vi "KickSkillVSS.vi"(8 "error in (no error)":errorcluster, 9 "BallRef":refnum<class "Ball.lvclass">, 10 "Robot":refnum<class "Robot.lvclass">, 11 "KickSkillVSS in":refnum<class "KickSkillVSS.lvclass">) -> (0 "error out":errorcluster, 2 "Robot out":refnum<class "Robot.lvclass">, 3 "KickSkillVSS out":refnum<class "KickSkillVSS.lvclass">)   [LabVIEW 2020, in "KickSkillVSS.lvclass"]
uses:
  KickSkillVSS.lvclass
  Robot_class/Robot.lvclass
  Ball_class/Ball.lvclass
  Field_class/Field.lvclass
  Utilities_class/Utilities.lvclass
  Object_class/Object.lvclass/Object.ctl
  Ball_class/Ball.lvclass/Ball.ctl
  Robot_class/Robot.lvclass/Robot.ctl
  Object_class/Read x.vi
  Object_class/Read y.vi
  Ball_class/Read v_x.vi
  Ball_class/Read v_y.vi
  Object_class/Read pos_est_x.vi
  Object_class/Read pos_est_y.vi
  Robot_class/Write orientation.vi
panel:
  in  "Field":refnum<class "Field.lvclass">
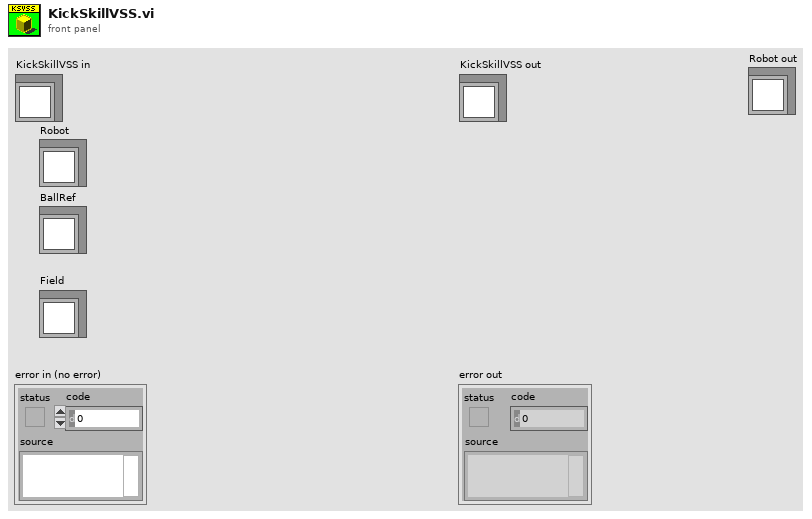
[diagram p1: front panel]
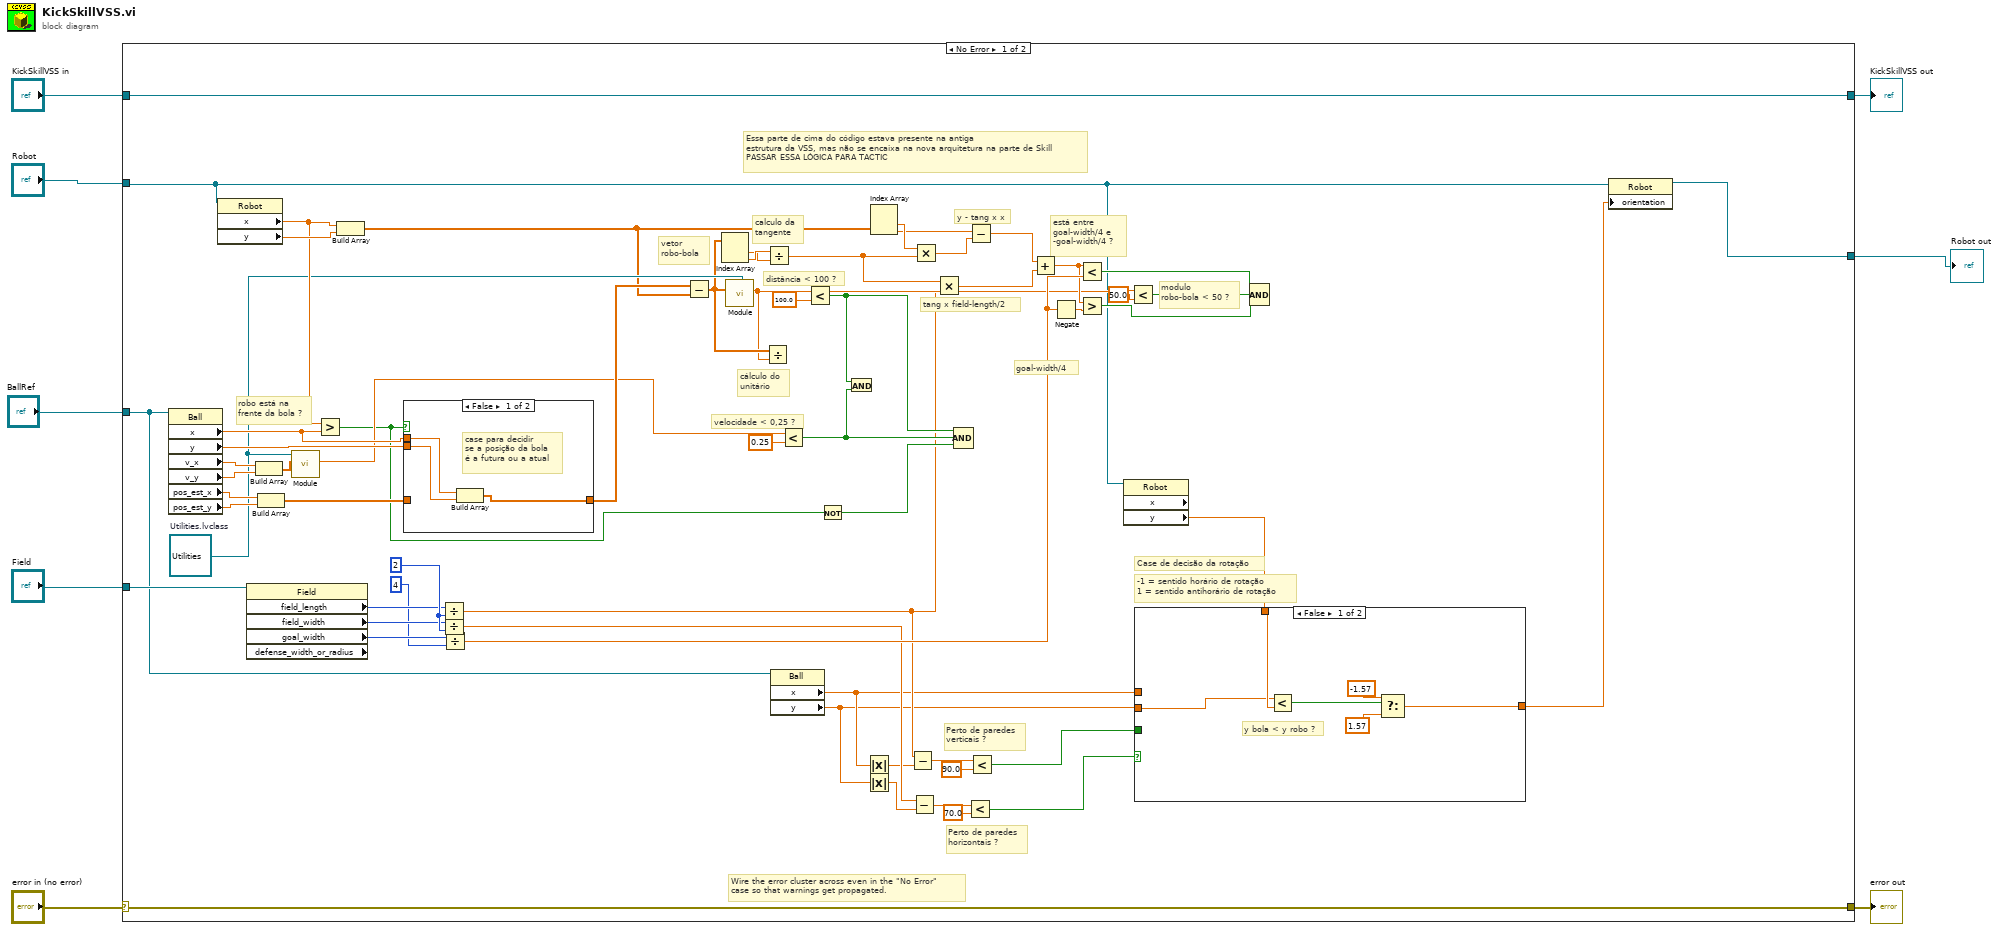
[diagram p0: block diagram]
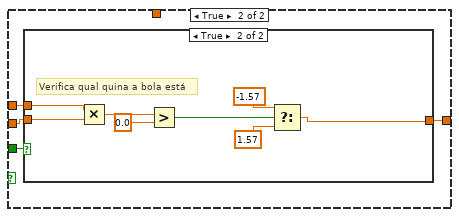
[diagram p2: hidden frame]
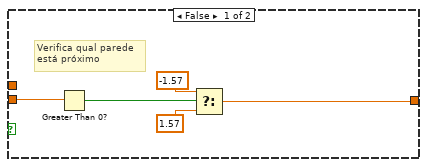
[diagram p3: hidden frame]
diagram:
  n1 = case shown="No Error" "error in (no error)" {
    selector: "error in (no error)" -> [w69 w100]
    tunnel: [w69 w100] -> w7
    tunnel: [w70 w99] -> w5
    tunnel: "KickSkillVSS in" -> [w70 w99]
    tunnel: "Robot" -> [w10 w98]
    tunnel: [w68 w98] -> w3
    tunnel: "BallRef" -> [w24 _]
    tunnel: "Field" -> [w49 _]
    frame No Error {
      w42 = 2
      w56 = refnum<class "Utilities.lvclass"> refnum  # Utilities.lvclass
      # "Essa parte de cima do código estava presente na antiga \nestrutura da VSS, mas não se encaixa na nova arquitetura na parte de Skill\nPASSAR ESSA LÓGICA PARA TACTIC"
      # "-1 = sentido horário de rotação\n1 = sentido antihorário de rotação"
      # "Case de decisão da rotação"
      # "Perto de paredes\nhorizontais ?"
      # "Perto de paredes\nverticais ?"
      # "modulo\nrobo-bola < 50 ?"
      # "está entre\ngoal-width/4 e\n-goal-width/4 ?"
      # "goal-width/4"
      # "y - tang x x"
      # "tang x field-length/2"
      # "velocidade < 0,25 ?"
      # "distância < 100 ?"
      # "cálculo do\nunitário"
      # "calculo da\ntangente"
      # "vetor \nrobo-bola"
      # "robo está na\nfrente da bola ?"
      # "Wire the error cluster across even in the \"No Error\"\ncase so that warnings get propagated."
      n2 = property class="Ball"(reference=w24) -> ("x"=w57:dbl, "y"=w58:dbl, "v_x"=w67:dbl, "v_y"=w66:dbl, "pos_est_x"=w64:dbl, "pos_est_y"=w63:dbl)  [unwired: 1 in, 2 out]
      n3 = property class="Robot"(reference=w10) -> ("x"=w61:dbl, "y"=w62:dbl)  [unwired: 1 in, 2 out]
      n4 = property class="Field" props=["field_length", "field_width", "goal_width", "defense_width_or_radius"](reference=w49) -> ("field_length"=w41:i32, "field_width"=w40:i32, "goal_width"=w34:i32)  [unwired: 1 in, 3 out]
      n5 = Build Array(w67, w66) -> (w65:dbl[])
      n6 = Build Array(w64, w63) -> (w59:dbl[])
      n7 = call-dynamic "Module.vi"("2D vector"=w65, "Utilities in"=w56) -> ("Modulo"=w50:dbl)  [unwired: 7 in, 2 out]
      n8 = Greater?(x=w61, y=w57) -> (0:w47:bool)
      n9 = Build Array(w61, w62) -> (w48:dbl[])
      n10 = case shown="False" w47 {
        tunnel: [w94 w97] -> w60
        tunnel: w59 -> [_ w97]
        tunnel: w58 -> [w96 _]
        tunnel: w57 -> [w95 _]
        frame False {
          # "case para decidir \nse a posição da bola \né a futura ou a atual"
          n11 = Build Array(w95, w96) -> (w94:dbl[])
        }
        frame True {
        }
      }
      n12 = Divide(x=w41, y=w42) -> (x/y=w21:dbl)
      n13 = Divide(x=w40, y=w42) -> (x/y=w23:dbl)
      n14 = Divide(x=w34, y=4) -> (x/y=w32:dbl)
      n15 = Subtract(x=w60, y=w48) -> (x-y=w53:dbl[])
      n16 = Index Array(array=w53) -> (element #1=w54:dbl, element #2=w55:dbl)  [unwired: 2 in]
      n17 = call-dynamic "Module.vi"("2D vector"=w53, "Utilities in"=w56) -> ("Modulo"=w28:dbl)  [unwired: 7 in, 2 out]
      n18 = Divide(x=w53, y=w28) -> ()  [unwired: 1 out]
      n19 = Divide(x=w55, y=w54) -> (x/y=w43:dbl)
      n20 = property class="Ball"(reference=w24) -> ("x"=w13:dbl, "y"=w12:dbl)  [unwired: 1 in, 2 out]
      n21 = Less?(x=w50, y=0.25) -> (x < y?=w45:bool)
      n22 = Less?(x=w28, y=100.0) -> (x < y?=w46:bool)
      n23 = Not(x=w47) -> (.not. x?=w44:bool)
      n24 = And(x=w46, y=w45) -> ()  [unwired: 1 out]
      n25 = Absolute Value(x=w13) -> (abs(x)=w20:dbl)
      n26 = Absolute Value(x=w12) -> (abs(x)=w22:dbl)
      n27 = Index Array(array=w48) -> (element #1=w39:dbl, element #2=w38:dbl)  [unwired: 2 in]
      n28 = Subtract(x=w21, y=w20) -> (x-y=w19:dbl)
      n29 = Subtract(x=w23, y=w22) -> (x-y=w18:dbl)
      n30 = Multiply(x=w39, y=w43) -> (x*y=w37:dbl)
      n31 = Multiply(x=w43, y=w21) -> (x*y=w35:dbl)
      n32 = Compound Arithmetic op=AND(w46, w45, w44) -> ()  [unwired: 1 out]
      n33 = Less?(x=w18, y=70.0) -> (x < y?=w15:bool)
      n34 = Subtract(x=w38, y=w37) -> (x-y=w36:dbl)
      n35 = Less?(x=w19, y=90.0) -> (x < y?=w14:bool)
      n36 = Add(x=w36, y=w35) -> (x+y=w30:dbl)
      n37 = Negate(x=w32) -> (-x=w31:dbl)
      n38 = Less?(x=w30, y=w32) -> (x < y?=w26:bool)
      n39 = Greater?(x=w30, y=w31) -> (0:w25:bool)
      n40 = property class="Robot" props=["x", "y"](reference=w10) -> ("y"=w9:dbl)  [unwired: 1 in, 3 out]
      n41 = Less?(x=w28, y=50.0) -> (x < y?=w27:bool)
      n42 = case shown="False" w15 {
        tunnel: w14 -> [_ w80]
        tunnel: w13 -> [_ w79]
        tunnel: w12 -> [w72 w78]
        tunnel: [w71 w77] -> w11
        tunnel: w9 -> [w73 _]
        frame False {
          # "y bola < y robo ?"
          n43 = Less?(x=w72, y=w73) -> (x < y?=w74:bool)
          n44 = Select(t=-1.57, s=w74, f=1.57) -> (s? t:f=w71:dbl)
        }
        frame True {
          n45 = case shown="True" w80 {
            tunnel: w79 -> [_ w93]
            tunnel: w78 -> [w85 w92]
            tunnel: [w81 w86] -> w77
            frame False {
              # "Verifica qual parede \nestá próximo"
              n46 = Greater Than 0?(x=w85) -> (x > 0?=w82:bool)
              n47 = Select(t=-1.57, s=w82, f=1.57) -> (s? t:f=w81:dbl)
            }
            frame True {
              # "Verifica qual quina a bola está"
              n48 = Multiply(x=w93, y=w92) -> (x*y=w90:dbl)
              n49 = Greater?(x=w90, y=0.0) -> (0:w89:bool)
              n50 = Select(t=-1.57, s=w89, f=1.57) -> (s? t:f=w86:dbl)
            }
          }
        }
      }
      n51 = Compound Arithmetic op=AND(w26, w27, w25) -> ()  [unwired: 1 out]
      n52 = property class="Robot"(reference=w10, "orientation"=w11) -> (reference out=w68:refnum<class "Robot.lvclass">)  [unwired: 1 in, 1 out]
    }
    frame Error {
    }
  }
  "error out" <- w7
  "KickSkillVSS out" <- w5
  "Robot out" <- w3
